vi "SetLocalMode.vi"(8 "error in (no error)":errorcluster, 10 "Front Panel Mode":bool=TRUE caption="Front Panel Mode (T = Local)", 11 "DigitalOutput_Simulation In":refnum<class "TesteractHAL_DigitalOutput_Simulation.lvclass">) -> (0 "error out":errorcluster, 3 "DigitalOutput_Simulation Out":refnum<class "TesteractHAL_DigitalOutput_Simulation.lvclass">)   [LabVIEW 2017, in "TesteractHAL_DigitalOutput_Simulation.lvlib" / "TesteractHAL_DigitalOutput_Simulation.lvclass"]
uses:
  TesteractHAL_DigitalOutput_Simulation.lvclass
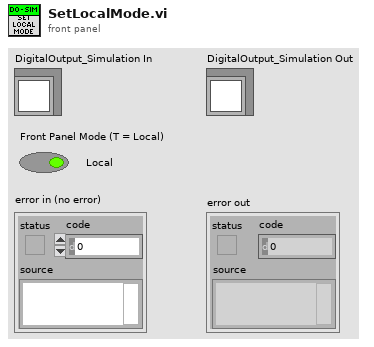
[diagram p1: front panel]
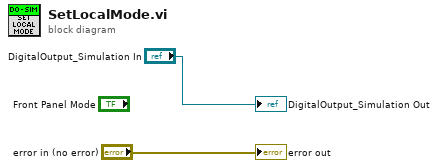
[diagram p0: block diagram]
diagram:
  "error out" <- "error in (no error)"
  "DigitalOutput_Simulation Out" <- "DigitalOutput_Simulation In"
